vi "FT_Set_USB_Parameters.vi"(1 "In Transfer Size":u32=65536, 2 "Handle":u32) -> (0 "FT_Status":u32(ring) items=["FT_OK", "FT_INVALID_HANDLE", "FT_DEVICE_NOT_FOUND", "FT_DEVICE_NOT_OPENED", "FT_IO_ERROR", "FT_INSUFFICIENT_RESOURCES", "FT_INVALID_PARAMETER", "FT_INVALID_BAUD_RATE", "FT_DEVICE_NOT_OPENED_FOR_ERASE", "FT_DEVICE_NOT_OPENED_FOR_WRITE", "FT_FAILED_TO_WRITE_DEVICE", "FT_EEPROM_READ_FAILED", "FT_EEPROM_WRITE_FAILED", "FT_EEPROM_ERASE_FAILED", "FT_EEPROM_NOT_PRESENT", "FT_EEPROM_NOT_PROGRAMMED", "FT_INVALID_ARGS", "FT_NOT_SUPPORTED", "FT_OTHER_ERROR"])   [LabVIEW 2013, in "DDS9954_v2013.lvlib"]
uses:
  DDS9954_v2013.lvlib
  ftd2xx.dll
panel:
  in  "Out Transfer Size":u32
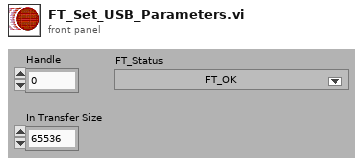
[diagram p1: front panel]
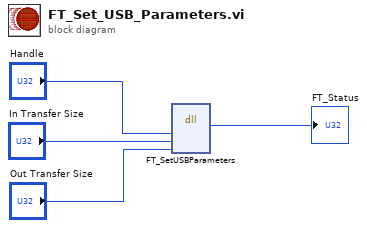
[diagram p0: block diagram]
diagram:
  n1 = dll-call lib="E:/Users/Disorder-Rb-Control/Documents/gitRepos/SetList/codes/DeviceVIs/DDS/ftd2xx.dll" fn="FT_SetUSBParameters"("Handle"="Handle", "InTransferSize"="In Transfer Size", "OutTransferSize"="Out Transfer Size") -> ("FT_Status"=→"FT_Status":u32)  [unwired: 6 in, 2 out]
